vi "GVZeitZyklus.vi"() -> ()   [LabVIEW 2010]
panel:
  out "MethodenZeit":dbl
  out "BigBen":dbl
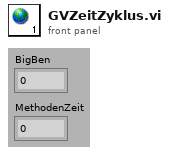
[diagram p1: front panel]
diagram:
